vi "MALT40IO get one input.vi"() -> ()   [LabVIEW 2018]
uses:
  <instrlib>/AltonTech MALT/AltonTech MALT200817.lvlib
panel:
  in  "DIn":i32=1
  in  "Address":i32=3 format="%02x"
  out "status":bool
  in  "stop":bool
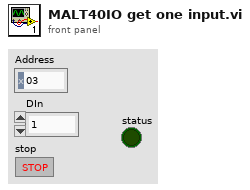
[diagram p1: front panel]
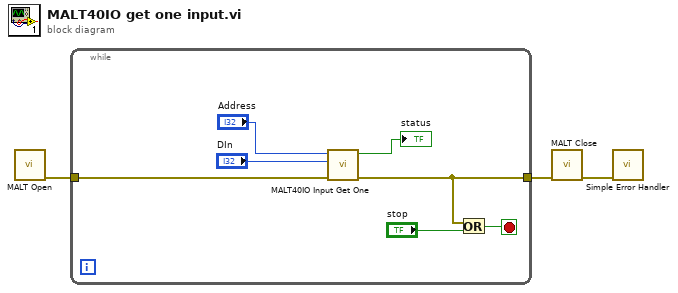
[diagram p0: block diagram]
diagram:
  n1 = call <instrlib>:"MALT Open.vi"() -> ("error out"=w3:errorcluster)  [unwired: 10 in, 1 out]
  n2 = while {
    tunnel: w3 -> [w10]
    tunnel: [w6] -> w2
    stop <- w8 stop-if-true
    n3 = call <instrlib>:"MALT40IO Input Get One.vi"("error in"=w10, "Port"="DIn", "Address"="Address") -> ("error out"=w6:errorcluster, "status"=→"status":bool)  [unwired: 7 in]
    n4 = Or(x=w6, y="stop") -> (x .or. y?=w8:bool)
  }
  n5 = call <instrlib>:"MALT Close.vi"("error in"=w2) -> ("error out"=w1:errorcluster)  [unwired: 10 in]
  n6 = call <vilib>:"Simple Error Handler.vi"("error in (no error)"=w1) -> ()  [unwired: 4 in, 5 out]
